vi "translate error response.vi"(11 "error responses":T3) -> (3 "fault handling":T1)   [LabVIEW 2013, in "Standard Engine Runtime.lvclass"]
doc: "Converts available error responses into an ordered array of actions."
uses:
  Standard Engine Runtime.lvclass
  error responses.ctl
  Configuration/error options.ctl
  main engine/fault handling spec.ctl
  Configuration/Error Actions.ctl
  Configuration/Standard Engine Configuration.lvclass
  main engine/main engine.lvlib
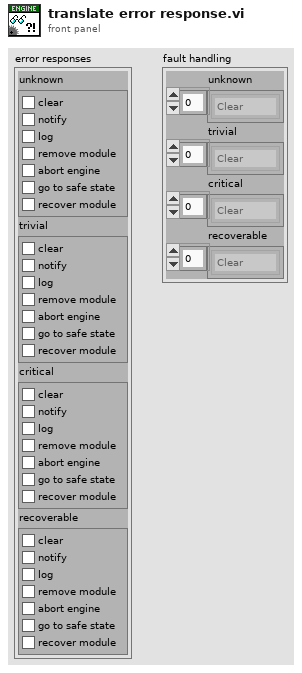
[diagram p1: front panel]
types:
  T1 = typedef "main engine.lvlib/fault handling spec.ctl" = cluster{"unknown":T2[], "trivial":T2[], "critical":T2[], "recoverable":T2[]}
  T2 = typedef "Standard Engine Configuration.lvclass/Error Actions.ctl" = enum16{"Clear", "Notify", "Log", "Stop Component", "Stop Engine", "Safe State", "Attempt Recovery"}
  T3 = typedef "Standard Engine Configuration.lvclass/error responses.ctl" = cluster{"unknown":T4, "trivial":T4, "critical":T4, "recoverable":T4}
  T4 = typedef "Standard Engine Configuration.lvclass/error options.ctl" = cluster{"clear":bool, "notify":bool, "log":bool, "remove module":bool, "abort engine":bool, "go to safe state":bool, "recover module":bool}
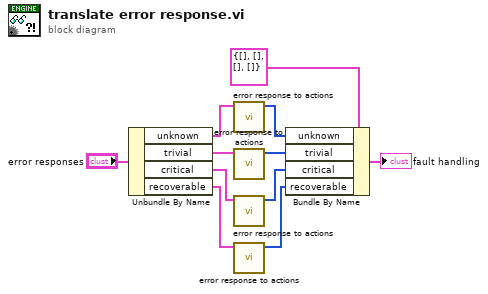
[diagram p0: block diagram]
diagram:
  n1 = Unbundle By Name("error responses") -> ("unknown"=w7:T4, "trivial"=w6:T4, "critical"=w1:T4, "recoverable"=w2:T4)
  n2 = call "error response to actions.vi"("error handling"=w7) -> ("actions"=w8:T2[])  [unwired: 10 in]
  n3 = call "error response to actions.vi"("error handling"=w6) -> ("actions"=w5:T2[])  [unwired: 10 in]
  n4 = call "error response to actions.vi"("error handling"=w1) -> ("actions"=w4:T2[])  [unwired: 10 in]
  n5 = call "error response to actions.vi"("error handling"=w2) -> ("actions"=w3:T2[])  [unwired: 10 in]
  n6 = Bundle By Name(cluster=T1 {"unknown"=[], "trivial"=[], "critical"=[], "recoverable"=[]} ("fault handling"), "unknown"=w8, "trivial"=w5, "critical"=w4, "recoverable"=w3) -> (→"fault handling":T1)
